vi "manage measurement.vi"(7 "exp exec in":T1={"data file"={"autosave"=FALSE, "File refnum"=refnum, "data file path"=path ""}, "T log file"={"File refnum"=refnum, "T log file path"=path "", "exists"=FALSE}, "exp seq"={"wave params"={"Num of avg"=0, "Num points"=0, "Meas rate (Hz)"=0.0}, "Setpoints"=[], "#"=0, "index"=0, "elapsed time (s)"=0.0, "set time (s)"=0.0, "min settle (s)"=30.0, " Exec Status"=enum."Settling"}, "error"={"status"=FALSE, "code"=0, "source"=""}}) -> (8 "exp exec out":T1={"data file"={"autosave"=FALSE, "File refnum"=refnum, "data file path"=path ""}, "T log file"={"File refnum"=refnum, "T log file path"=path "", "exists"=FALSE}, "exp seq"={"wave params"={"Num of avg"=0, "Num points"=0, "Meas rate (Hz)"=0.0}, "Setpoints"=[], "#"=0, "index"=0, "elapsed time (s)"=0.0, "set time (s)"=0.0, "min settle (s)"=30.0, " Exec Status"=enum."Settling"}, "error"={"status"=FALSE, "code"=0, "source"=""}})   [LabVIEW 2019]
doc: "This subVI manages the measurmenent of the RC decay in the bug experiment.\n\nPaul K Dixon\nP3600\nCSUSB Physics"
uses:
  typedefs/PID exec cluster.ctl
  typedefs/data file info.ctl
  typedefs/bug temp file info.ctl
  typedefs/exp seq cluster.ctl
  typedefs/wvfm acq params.ctl
  typedefs/bug meas status.ctl
  typedefs/result.ctl
  typedefs/cap fit params.ctl
  typedefs/temp mode enum.ctl
  globals/Bug globals.vi
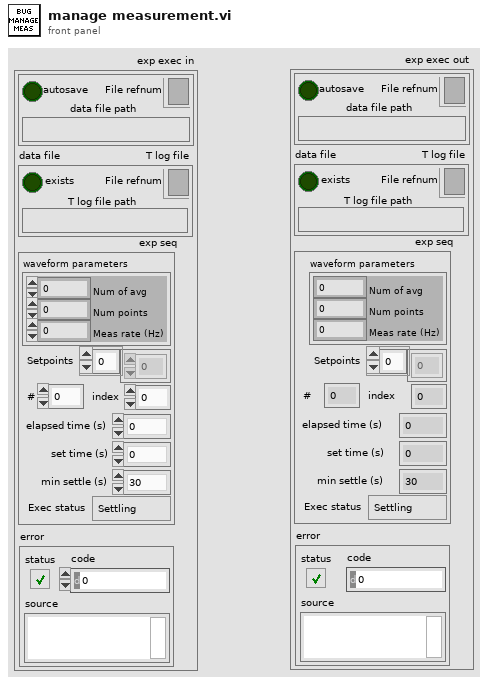
[diagram p1: front panel]
types:
  T1 = typedef "PID exec cluster.ctl" = cluster{"data file":T2, "T log file":T3, "exp seq":T4, "error":errorcluster}
  T2 = typedef "data file info.ctl" = cluster{"autosave":bool, "File refnum":refnum<file>, "data file path":path}
  T3 = typedef "bug temp file info.ctl" = cluster{"File refnum":refnum<file>, "T log file path":path, "exists":bool}
  T4 = typedef "exp seq cluster.ctl" = cluster{"wave params":T5, "Setpoints":dbl[], "#":i32, "index":i32, "elapsed time (s)":dbl, "set time (s)":dbl, "min settle (s)":dbl, " Exec Status":T6}
  T5 = typedef "wvfm acq params.ctl" = cluster{"Num of avg":i32, "Num points":i32, "Meas rate (Hz)":dbl}
  T6 = typedef "bug meas status.ctl" = enum32{"Settling", "Measuring", "Holding", "Exit"}
  T7 = typedef "result.ctl" = cluster{"Temp (C)":dbl, "RC Fit":T8, "wave":waveform(dbl), "Time (s)":dbl}
  T8 = typedef "cap fit params.ctl" = cluster{"Resistance (Ohms)":dbl, "Est Time constant (s)":dbl, "Est Capacitance (F)":dbl}
  T9 = typedef "temp cont cluster.ctl" = cluster{"T exec":T10, "T status":T12, "T params":T14, "utility":T15}
  T10 = typedef "temp exec cluster.ctl" = cluster{"T mode":T11, "exec setpoint":dbl, "reset":bool, "man power":dbl, "man":bool, "log":bool, "clear":bool}
  T11 = typedef "temp mode enum.ctl" = enum16{"settling", "measuring", "holding", "Exit"}
  T12 = typedef "temp indicator.ctl" = cluster{"Control status":T13, "Temp":dbl, "Power":dbl, "Time in settle band":dbl, "Settled":bool, "Low":bool, "High":bool, "Setpoint":dbl, "Control":bool, "In Settle Band":bool}
  T13 = typedef "temp control status.ctl" = enum16{"In Settle Band", "In Control Band", "Below Control Band", "Above Control Band"}
  T14 = typedef "PID control parameters.ctl" = cluster{"Setpoint":dbl, "Control Bandwidth":dbl, "Integral Time":dbl, "Int\nON":bool, "Derivative Tme":dbl, "Der\nON":bool, "Settle Bandwidth":dbl, "Settle Time":dbl}
  T15 = typedef "temp cont utility.ctl" = cluster{"meas index":i32, "wait (ms)":i32, "H Vmax":dbl, "power out":dbl, "heat volt out":dbl, "heat volt in":dbl, "therm volt":dbl, "t T P hist":dbl[][], "cont hist":dbl[][]}
  T16 = typedef "measurement.ctl" = cluster{"wvfm params":T5, "avg":waveform(dbl), "raw wvfms":waveform(dbl)[], "progress":cluster{"avg done":bool, "meas index":i32, "N waves":i32}, "t (s)":dbl}
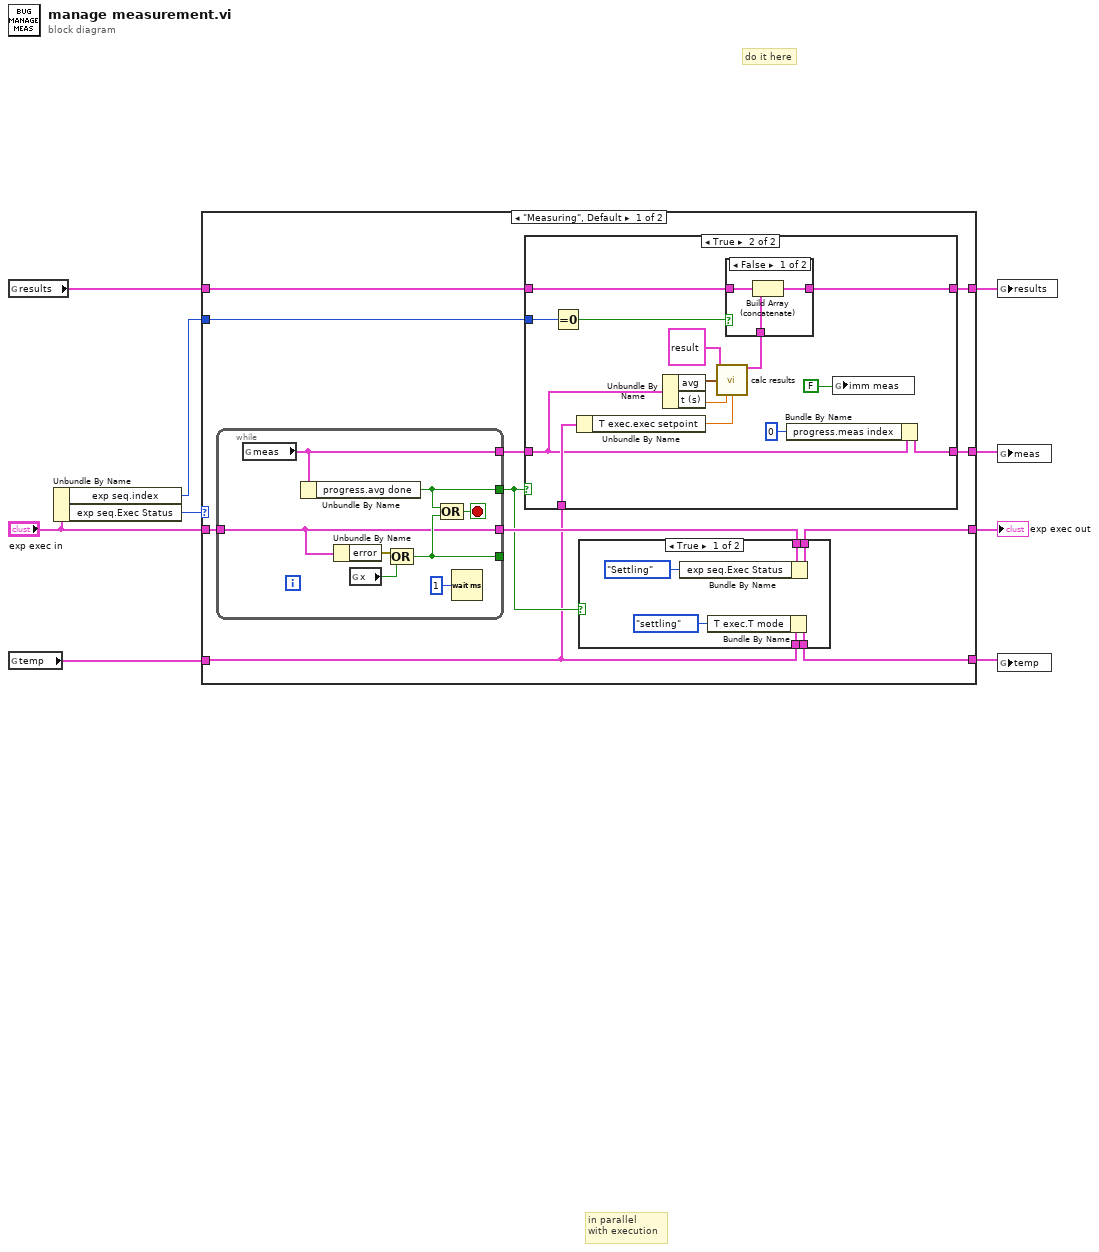
[diagram p0: block diagram]
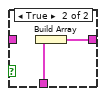
[diagram p3: hidden frame]
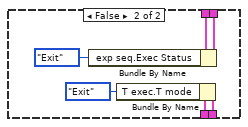
[diagram p4: hidden frame]
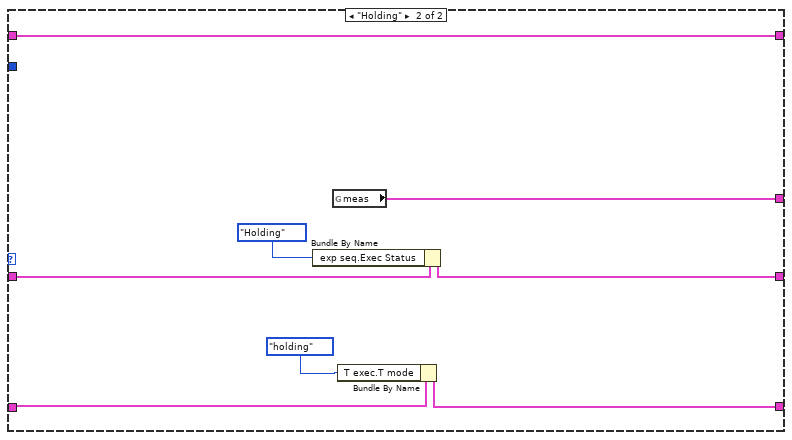
[diagram p5: hidden frame]
diagram:
  # "do it here"
  # "in parallel\nwith execution"
  n1 = global read "Bug globals.vi" "results"() -> (w3:T7[])
  n2 = global read "Bug globals.vi" "temp"() -> (w9:T9)
  n3 = Unbundle By Name("exp exec in") -> ("exp seq.index"=w1:i32, "exp seq.Exec Status"=w8:T6)
  n4 = case shown="\"Measuring\", Default" w8 {
    tunnel: w9 -> [w11 w66]
    tunnel: [w19 w63] -> w6
    tunnel: [w12 w65] -> w5
    tunnel: "exp exec in" -> [w18 w64]
    tunnel: [w17 w62] -> w4
    tunnel: w3 -> [w15 w69]
    tunnel: [w14 w69] -> w2
    tunnel: w1 -> [w13 _]
    frame "Measuring", Default {
      n5 = while {
        tunnel: [w59] -> _
        tunnel: [w58] -> w16
        tunnel: [w56] -> w10
        tunnel: w18 -> [w57]
        tunnel: [w57] -> w20
        stop <- w60 stop-if-true
        n6 = global read "Bug globals.vi" "meas"() -> (w56:T16)
        n7 = Unbundle By Name(w56) -> ("progress.avg done"=w58:bool)
        n8 = Unbundle By Name(w57) -> ("error"=w61:errorcluster)
        n9 = global read "Bug globals.vi" "x"() -> (w55:bool)
        n10 = Compound Arithmetic op=OR(w61, w55) -> (w59:bool)
        n11 = Compound Arithmetic op=OR(w58, w59) -> (w60:bool)
        n12 = Wait (ms)(milliseconds to wait=u32 1) -> ()  [unwired: 1 out]
      }
      n13 = case shown="True" w16 {
        tunnel: w10 -> [w22 w26]
        tunnel: [w22 w28] -> w17
        tunnel: w15 -> [w21 w32]
        tunnel: [w21 w29] -> w14
        tunnel: w13 -> [_ w27]
        tunnel: w11 -> [_ w35]
        frame False {
        }
        frame True {
          n14 = Equal To 0?(x=w27) -> (x = 0?=w31:bool)
          n15 = Unbundle By Name(w35) -> ("T exec.exec setpoint"=w34:dbl)
          n16 = Unbundle By Name(w26) -> ("avg"=w36:waveform(dbl), "t (s)"=w24:dbl)
          n17 = call "calc results.vi"("result in"=T7 {"Temp (C)"=0.0, "RC Fit"={"Resistance (Ohms)"=100000.0, "Est Time constant (s)"=0.0, "Est Capacitance (F)"=0.0}, "wave"={"t0"=timestamp(0 s since 1904-01-01), "dt"=1.0, "Y"=[]}, "Time (s)"=0.0} ("result"), "avg"=w36, "time (s)"=w24, "exec setpoint"=w34) -> ("result out"=w30:T7)  [unwired: 11 in]
          n18 = case shown="False" w31 {
            tunnel: w32 -> [w39 _]
            tunnel: w30 -> [w38 w41]
            tunnel: [w37 w40] -> w29
            frame False {
              n19 = Build Array (concatenate)(w39, w38) -> (w37:T7[])
            }
            frame True {
              n20 = Build Array(w41) -> (w40:T7[])
            }
          }
          n21 = Bundle By Name(cluster=w26, "progress.meas index"=0) -> (w28:T16)
          n22 = global write "Bug globals.vi" "imm meas"(FALSE ("imm meas")) -> ()
        }
      }
      n23 = case shown="True" w16 {
        tunnel: w20 -> [w47 w53]
        tunnel: [w46 w52] -> w19
        tunnel: w11 -> [w44 w50]
        tunnel: [w42 w48] -> w12
        frame True {
          n24 = Bundle By Name(cluster=w47, "exp seq.Exec Status"=bug_meas_status."Settling" ("exp seq. Exec Status")) -> (w46:T1)
          n25 = Bundle By Name(cluster=w44, "T exec.T mode"=temp_mode_enum."settling") -> (w42:T9)
        }
        frame False {
          n26 = Bundle By Name(cluster=w53, "exp seq.Exec Status"=bug_meas_status."Exit" ("exp seq. Exec Status")) -> (w52:T1)
          n27 = Bundle By Name(cluster=w50, "T exec.T mode"=temp_mode_enum."Exit") -> (w48:T9)
        }
      }
    }
    frame "Holding" {
      n28 = Bundle By Name(cluster=w64, "exp seq.Exec Status"=bug_meas_status."Holding" ("exp seq. Exec Status")) -> (w63:T1)
      n29 = global read "Bug globals.vi" "meas"() -> (w62:T16)
      n30 = Bundle By Name(cluster=w66, "T exec.T mode"=temp_mode_enum."holding") -> (w65:T9)
    }
  }
  "exp exec out" <- w6
  n31 = global write "Bug globals.vi" "results"(w2) -> ()
  n32 = global write "Bug globals.vi" "meas"(w4) -> ()
  n33 = global write "Bug globals.vi" "temp"(w5) -> ()
